vi "GetAllTestStatus.vi"(11 "Model in":refnum<class "Model.lvclass">) -> (2 "AllTestStatus":T1, 3 "Model out":refnum<class "Model.lvclass">)   [LabVIEW 2016, in "Model.lvclass"]
uses:
  Model.lvclass
  Typedefs/AllTestStatus.ctl
  Typedefs/TestStatus.ctl
  Model.lvclass/Model.ctl
  Typedefs/HPMT_Typedefs.lvlib
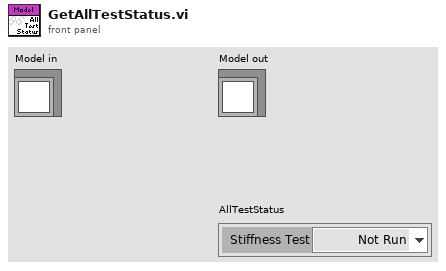
[diagram p1: front panel]
types:
  T1 = typedef "HPMT_Typedefs.lvlib/AllTestStatus.ctl" = cluster{"Stiffness Test":T2}
  T2 = typedef "HPMT_Typedefs.lvlib/TestStatus.ctl" = enum16{"Not Run", "Running", "Passed", "Failed"}
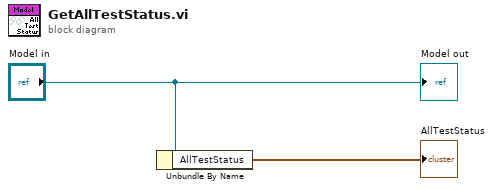
[diagram p0: block diagram]
diagram:
  n1 = Unbundle By Name("Model in") -> ("AllTestStatus"=→"AllTestStatus":T1)
  "Model out" <- "Model in"
